vi "IsPenalty.vi"(0 "object in":refnum<class "DefendGoalTactic.lvclass">, 1 "command_interpreted":T1=enum."Halt", 2 "pos(x, y) da bola":dbl[](array[numeric]), 5 "error in (no error)":errorcluster) -> (14 "object out":refnum<class "DefendGoalTactic.lvclass">, 16 "IsPenalty":bool, 19 "error out":errorcluster)   [LabVIEW 2024, in "DefendGoalTactic.lvclass"]
uses:
  DefendGoalTactic.lvclass
  Referee_class/command_interpreted.ctl
  <vilib>/Analysis/_algsub.llb/Real Vector Norm.vi
  <vilib>/Analysis/NI_AALPro.lvlib
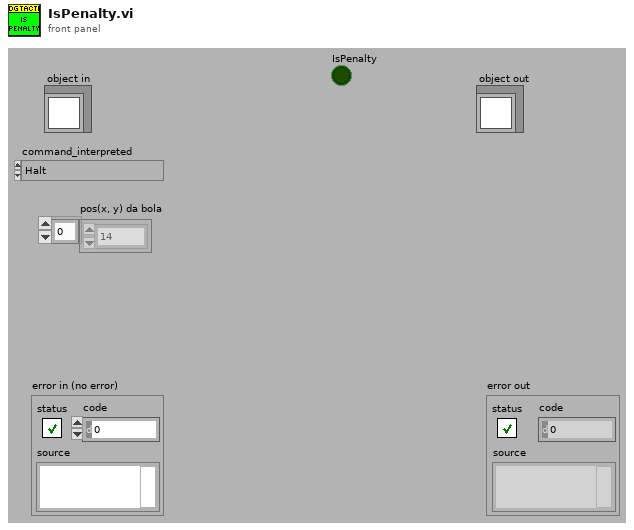
[diagram p1: front panel]
types:
  T1 = typedef "command_interpreted.ctl" = enum16{"Goal Ally", "Goal Enemy", "Ball Placement Enemy", "Ball Placement Ally", "Normal Half Time", "Extra Time  Break", "Extra Half Time", "None", "Post Game", "PKA Normal Start", "Prepare Kickoff Ally", "PKE Normal Start", "Prepare Kickoff Enemy", "Force Start", "Halt", "Timeout", "Prepare Penalty Ally", "Prepare Penalty Enemy", "PPA NormalStart", "PPE Normal Start", "Indirect Free Ally", "Direct Free Enemy", "Direct Free Ally", "Indirect Free Enemy", "Stop"}
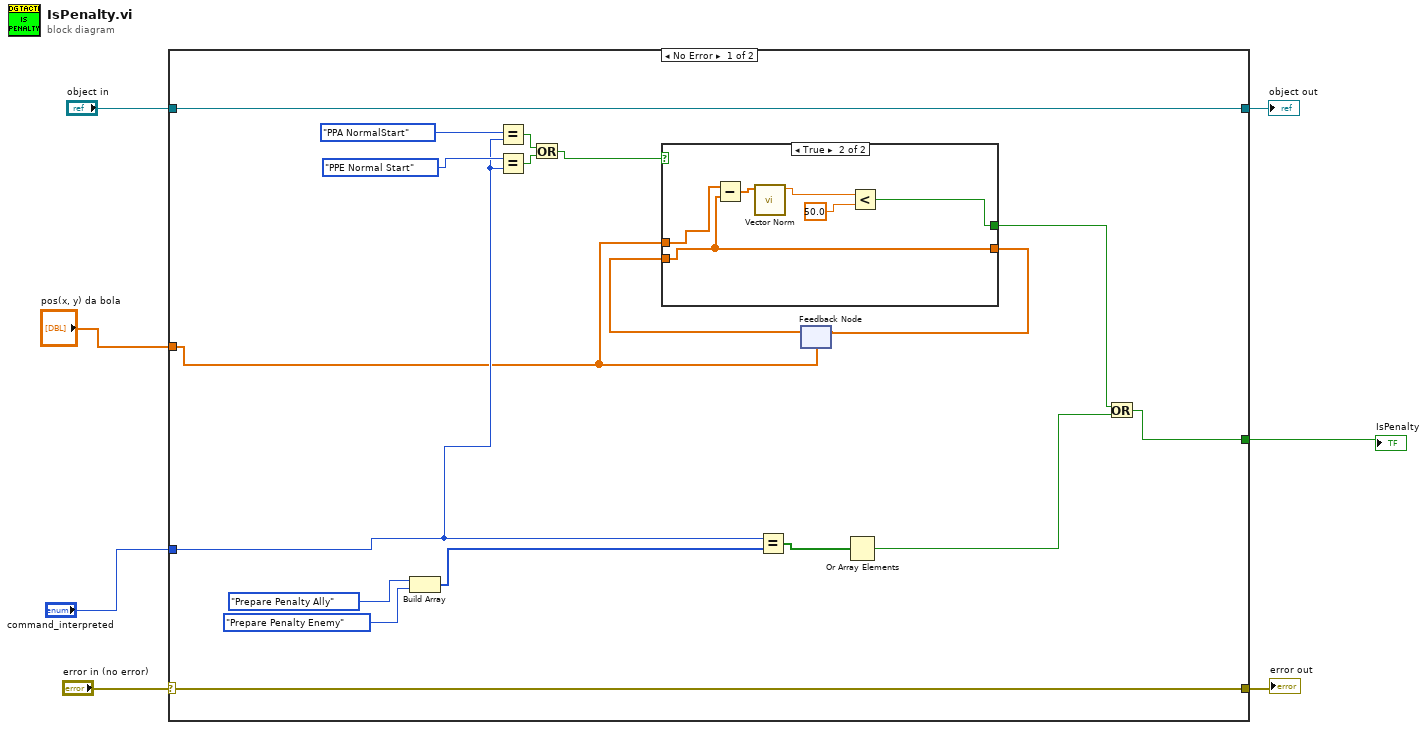
[diagram p0: block diagram]
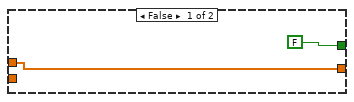
[diagram p2: hidden frame]
diagram:
  n1 = case shown="No Error" "error in (no error)" {
    selector: "error in (no error)" -> [w24 w35]
    tunnel: [w24 w35] -> w6
    tunnel: [w25 w34] -> w4
    tunnel: "object in" -> [w25 w34]
    tunnel: "command_interpreted" -> [w12 _]
    tunnel: [w8 _] -> w2
    tunnel: "pos(x, y) da bola" -> [w11 _]
    frame No Error {
      n2 = Build Array(command_interpreted."Prepare Penalty Ally" ("command_interpreted"), command_interpreted."Prepare Penalty Enemy" ("command_interpreted")) -> (w21:T1[])
      n3 = Equal?(x=command_interpreted."PPA NormalStart" ("command_interpreted"), y=w12) -> (x = y?=w15:bool)
      n4 = Equal?(x=command_interpreted."PPE Normal Start" ("command_interpreted"), y=w12) -> (x = y?=w14:bool)
      n5 = Or(x=w15, y=w14) -> (x .or. y?=w13:bool)
      n6 = Equal?(x=w12, y=w21) -> (x = y?=w20:bool[])
      n7 = feedback #1(w11) -> (w19:dbl[])
      n8 = case shown="True" w13 {
        tunnel: w19 -> [_ w31]
        tunnel: [w27 w31] -> w18
        tunnel: w11 -> [w27 w32]
        tunnel: [FALSE w33] -> w9
        frame False {
        }
        frame True {
          n9 = Subtract(x=w32, y=w31) -> (x-y=w29:dbl[])
          n10 = call-poly <vilib>:"Vector Norm.vi"("Input Vector"=w29) -> ("norm"=w28:dbl)  [unwired: 9 in, 1 out]
          n11 = Less?(x=w28, y=50.0) -> (x < y?=w33:bool)
        }
      }
      n12 = feedback-in #1(w18) -> ()
      n13 = Or Array Elements(Boolean array=w20) -> (logical OR=w10:bool)
      n14 = Or(x=w9, y=w10) -> (x .or. y?=w8:bool)
    }
    frame Error {
    }
  }
  "error out" <- w6
  "object out" <- w4
  "IsPenalty" <- w2
